vi "Find Case Structure From Event Structure.vi"(8 "error in (no error)":errorcluster, 11 "EvntStruct Refnum":refnum<vi>) -> (0 "error out":errorcluster, 2 "CaseStructure out":refnum<vi>)   [LabVIEW 2013, in "JKI State Machine API.lvlib" / "JKI SM.lvclass"]
uses:
  JKI SM.lvclass
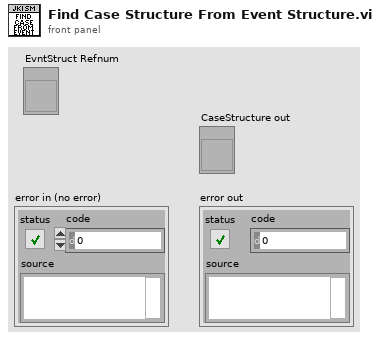
[diagram p1: front panel]
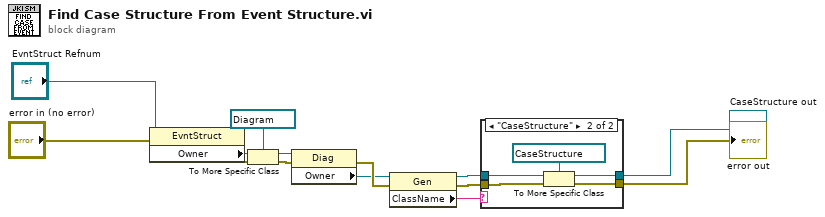
[diagram p0: block diagram]
diagram:
  n1 = property class="EvntStruct"(reference="EvntStruct Refnum", error in="error in (no error)") -> (error out=w6:errorcluster, "Owner"=w3:refnum<vi>)  [unwired: 1 out]
  n2 = To More Specific Class(target class=refnum<vi> refnum ("Diag Refnum"), reference=w3, error in=w6) -> (specific class reference=w7:refnum<vi>, error out=w5:errorcluster)
  n3 = property class="Diag"(reference=w7, error in=w5) -> (error out=w12:errorcluster, "Owner"=w10:refnum<vi>)  [unwired: 1 out]
  n4 = property class="Gen"(reference=w10, error in=w12) -> (reference out=w11:refnum<vi>, error out=w13:errorcluster, "ClassName"=w14:string)
  n5 = case shown="\"CaseStructure\"" w14 {
    tunnel: [_ w19] -> w8
    tunnel: [w15 w18] -> w9
    tunnel: w11 -> [_ w17]
    tunnel: w13 -> [w15 w16]
    frame Default {
    }
    frame "CaseStructure" {
      n6 = To More Specific Class(target class=refnum<vi> refnum ("CaseSel Refnum"), reference=w17, error in=w16) -> (specific class reference=w19:refnum<vi>, error out=w18:errorcluster)
    }
  }
  "error out" <- w9
  "CaseStructure out" <- w8
